vi "Excit_Setup_Wfm.vi"(7 "Excit Number":i32, 8 "error in":errorcluster, 9 "Excit Waveforms File Filter":string, 10 "Excit Waveforms Path":path, 11 "EXCIT Waveforms Inputs":T1={"Excit Form"=enum."Swift", "Amplitude"=100.0, "Start Frequency"=250.0, "End Frequency"=1000.0, "Duration"=800.0, "Sampling Frequency"=5.0, "Swift Factor"=0.5, "Chirp Apodisation"=3.5, "Amplitude 2"=100.0, "Start Frequency 2"=250.0, "End Frequency 2"=350.0} caption="EXCIT Inputs" {"End Frequency 2" min=1.0 max=10000.0; "Start Frequency 2" min=1.0 max=10000.0; "Amplitude 2" min=1.0 max=100.0; "Chirp Apodisation" min=1.0 max=5.0 step=0.1; "Swift Factor" min=0.1 max=3.0 step=0.1; "Sampling Frequency" min=10.0 max=100.0 step=1.0; "Duration" min=1.0 max=1000000.0 step=1.0; "End Frequency" min=1.0 max=10000.0; "Start Frequency" min=1.0 max=10000.0 step=0.1; "Amplitude" min=1.0 max=100.0}) -> (0 "error out":errorcluster caption="sortie d'erreur", 2 "EXCIT Waveforms Inputs":T1={"Excit Form"=enum."Swift", "Amplitude"=100.0, "Start Frequency"=250.0, "End Frequency"=1000.0, "Duration"=800.0, "Sampling Frequency"=5.0, "Swift Factor"=0.5, "Chirp Apodisation"=3.5, "Amplitude 2"=100.0, "Start Frequency 2"=250.0, "End Frequency 2"=350.0} caption="EXCIT Inputs" {"End Frequency 2" min=1.0 max=10000.0; "Start Frequency 2" min=1.0 max=10000.0; "Amplitude 2" min=1.0 max=100.0; "Chirp Apodisation" min=1.0 max=5.0 step=0.1; "Swift Factor" min=0.1 max=3.0 step=0.1; "Sampling Frequency" min=10.0 max=100.0 step=1.0; "Duration" min=1.0 max=1000000.0 step=1.0; "End Frequency" min=1.0 max=10000.0; "Start Frequency" min=1.0 max=10000.0 step=0.1; "Amplitude" min=1.0 max=100.0}, 3 "Waveform Name":string)   [LabVIEW 2017]
doc: "From a start and end value, generates an adiabatic waveform signal of 2000 values (double).\nWrites this waveform into a binary file, in a big-endian format.\nDisplays the written data and the FFT of the signal.\nDefault Path for the generated file is D:\\PIRENEA\\EXCIT_WFMS\n\nAvailable Waveforms : Sinus, Swift, Chirp, Ramp (Up or Down), DoubleRamp (Up-Down or Down-Up)"
uses:
  controls/EXCIT_Waveforms_Inputs.ctl
  <vilib>/Analysis/NI_AALPro.lvlib
panel:
  out "Waveform Name":string
  in  "OK":bool
  out "Excitation FFT":cluster{dbl[], "Power Spectrum (V^2 rms)":dbl[]}(graph)
  out "Excitation Signal":T2(graph)
  out "FIFO used":i32
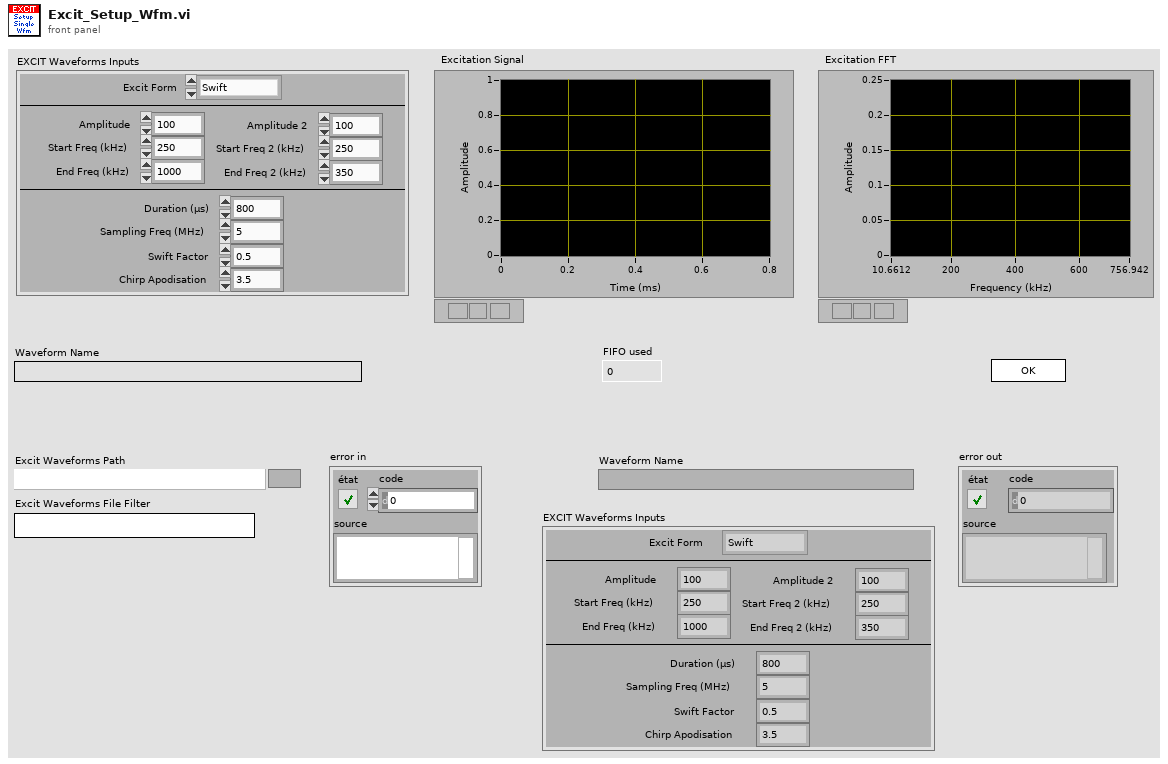
[diagram p1: front panel]
types:
  T1 = typedef "EXCIT_Waveforms_Inputs.ctl" = cluster{"Excit Form":enum16{"Sinus", "Chirp", "Swift", "TwoSwift", "Ramp"}, "Amplitude":dbl, "Start Frequency":dbl, "End Frequency":dbl, "Duration":dbl, "Sampling Frequency":dbl, "Swift Factor":dbl, "Chirp Apodisation":dbl, "Amplitude 2":dbl, "Start Frequency 2":dbl, "End Frequency 2":dbl}
  T2 = cluster{"X Time":dbl[], "Signal Excitation":dbl[]}
  T3 = enum16{"open", "replace", "create", "open or create", "replace or create", "replace or create with confirmation"}
  T4 = enum16{"big-endian, network order", "native, host order", "little-endian"}
  T5 = enum16{"Sinus", "Chirp", "Swift", "TwoSwift", "Ramp"}
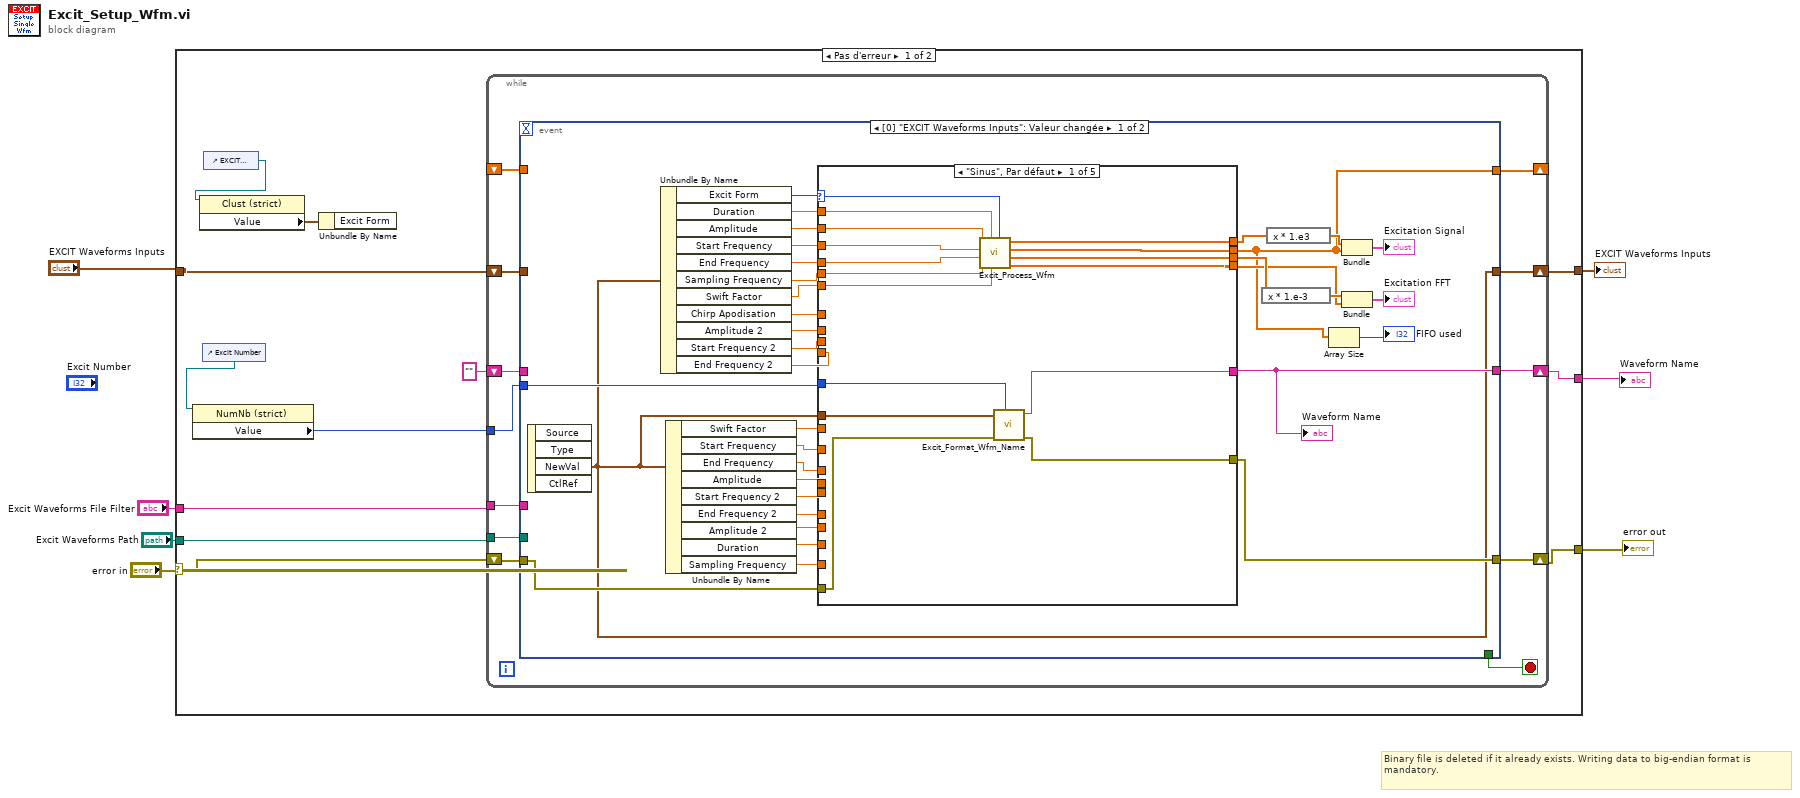
[diagram p0: block diagram]
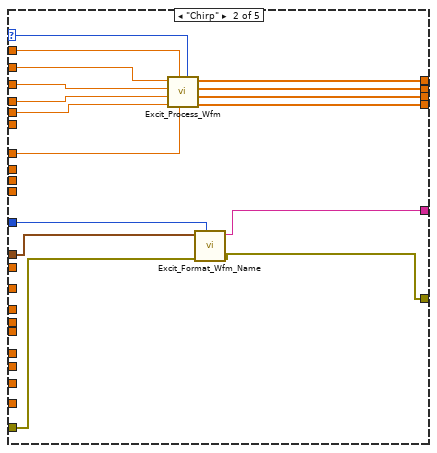
[diagram p2: hidden frame]
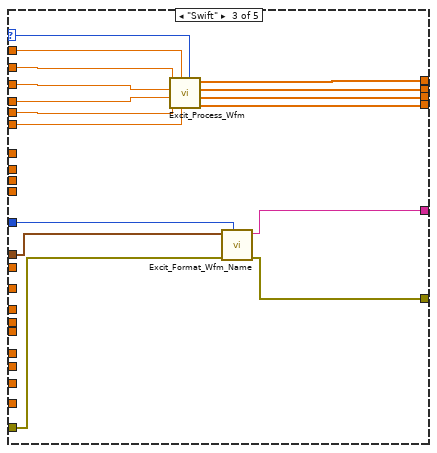
[diagram p3: hidden frame]
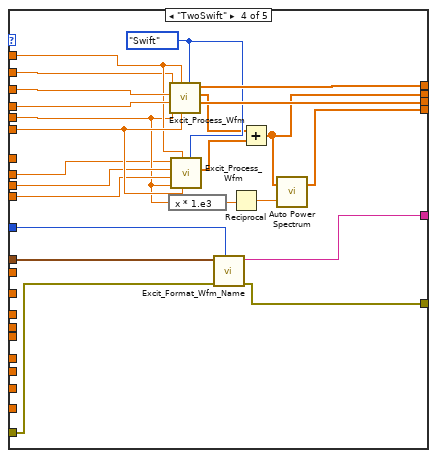
[diagram p4: hidden frame]
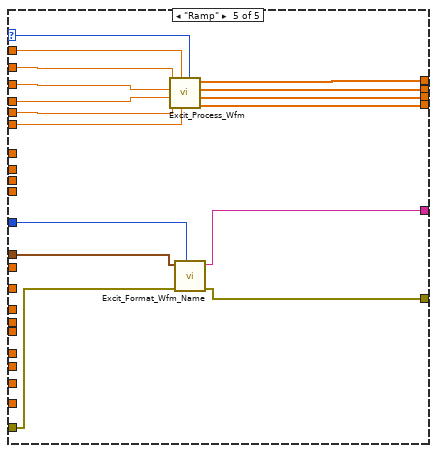
[diagram p5: hidden frame]
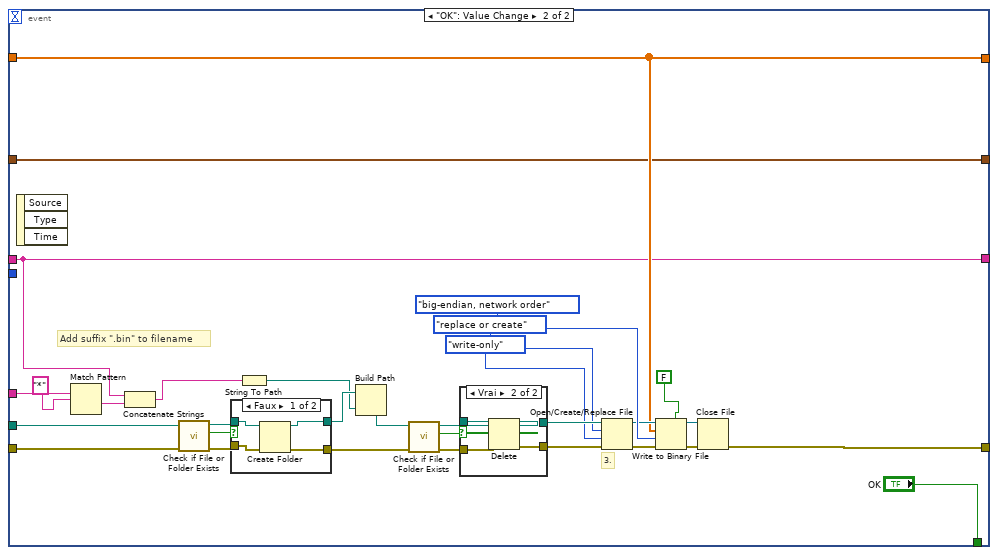
[diagram p6: hidden frame]
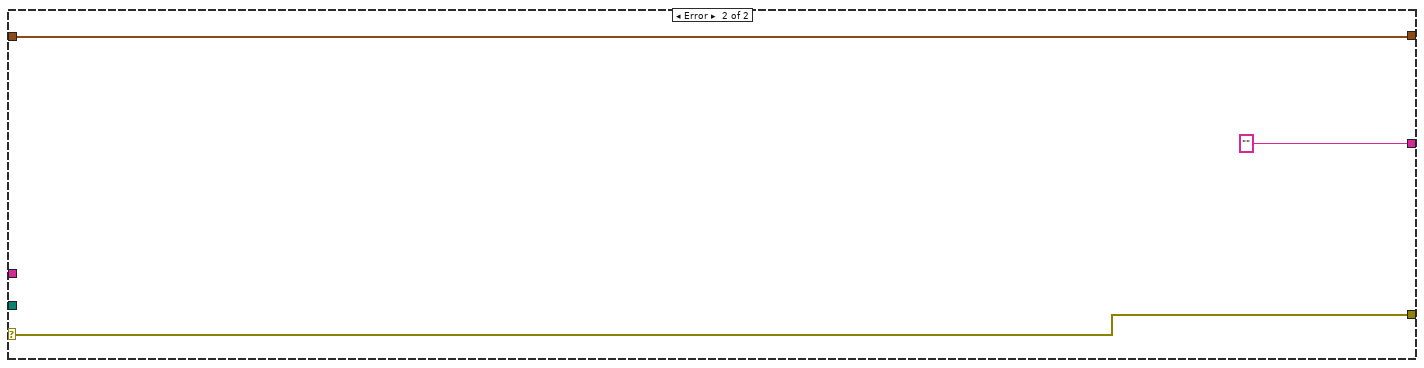
[diagram p9: hidden frame]
diagram:
  # "Binary file is deleted if it already exists. Writing data to big-endian format is mandatory."
  n1 = case shown="Pas d'erreur" "error in" {
    selector: "error in" -> [w10 w198]
    tunnel: [w19 w198] -> w7
    tunnel: "Excit Waveforms Path" -> [w18 _]
    tunnel: [w17 ""] -> w4
    tunnel: "Excit Waveforms File Filter" -> [w16 _]
    tunnel: "EXCIT Waveforms Inputs" -> [w14 w197]
    tunnel: [w13 w197] -> w1
    frame No Error {
      n2 = control-ref of="Excit Number"() -> (w12:refnum<vi>)
      n3 = property class="NumNb (strict)"(reference=w12) -> ("Value"=w11:i32)  [unwired: 1 in, 2 out]
      n4 = control-ref of="EXCIT Waveforms Inputs"() -> (w9:refnum<vi>)
      n5 = property class="Clust (strict)"(reference=w9) -> ("Value"=w8:T1)  [unwired: 1 in, 2 out]
      n6 = Unbundle By Name(w8) -> ()  [unwired: 1 out]
      n7 = while {
        tunnel: w18 -> [w25]
        shift-right: [w24] -> w19
        shift-left: w10 -> [w31]
        shift-right: [w29] -> _
        shift-left: _ -> [w27]
        shift-right: [w28] -> w17
        shift-left: "" -> [w26]
        tunnel: w16 -> [w23]
        shift-right: [w21] -> w13
        shift-left: w14 -> [w22]
        tunnel: w11 -> [w20]
        stop <- w30 stop-if-true
        n8 = event shown="[0] \"EXCIT Waveforms Inputs\": Valeur changée" {
          selector: _ -> [_ _]
          dyn-events: _ -> [_ _]
          timeout: _ -> [_ _]
          tunnel: [w36 w160] -> w24
          tunnel: w31 -> [w38 w162]
          tunnel: [_ "OK"] -> w30
          tunnel: [w37 w159] -> w29
          tunnel: [w35 w155] -> w28
          tunnel: w27 -> [_ w159]
          tunnel: w26 -> [_ w155]
          tunnel: w25 -> [_ w161]
          tunnel: w23 -> [_ w158]
          tunnel: w22 -> [_ w153]
          tunnel: [w32 w153] -> w21
          tunnel: w20 -> [w34 _]
          event Value Change {
            n9 = event-data() -> ("NewVal"=w32:T1)  [unwired: 1 in, 3 out]
            n10 = Unbundle By Name(w32) -> ("Excit Form"=w62:T5, "Duration"=w61:dbl, "Amplitude"=w60:dbl, "Start Frequency"=w59:dbl, "End Frequency"=w58:dbl, "Sampling Frequency"=w57:dbl, "Swift Factor"=w56:dbl, "Chirp Apodisation"=w55:dbl, "Amplitude 2"=w49:dbl, "Start Frequency 2"=w48:dbl, "End Frequency 2"=w47:dbl)
            n11 = Unbundle By Name(w32) -> ("Swift Factor"=w33:dbl, "Start Frequency"=w46:dbl, "End Frequency"=w45:dbl, "Amplitude"=w44:dbl, "Start Frequency 2"=w39:dbl, "End Frequency 2"=w43:dbl, "Amplitude 2"=w42:dbl, "Duration"=w41:dbl, "Sampling Frequency"=w40:dbl)
            n12 = case shown="\"Sinus\", Par défaut" w62 {
              selector: w62 -> [w80 w97 w107 _ w142]
              tunnel: w55 -> [_ w91 _ _ _]
              tunnel: w61 -> [w81 w96 w108 w122 w147]
              tunnel: w60 -> [w79 w95 w109 w120 w148]
              tunnel: w59 -> [w78 w94 w110 w126 w149]
              tunnel: w58 -> [w77 w93 w111 w125 w150]
              tunnel: w57 -> [w76 w92 w112 w121 w151]
              tunnel: w56 -> [w75 _ w113 w133 w152]
              tunnel: [w74 w90 w106 w136 w146] -> w54
              tunnel: [w73 w89 w105 w129 w145] -> w37
              tunnel: [w72 w88 w104 w135 w144] -> w52
              tunnel: [w71 w87 w103 w127 w143] -> w51
              tunnel: w49 -> [_ _ _ w119 _]
              tunnel: w48 -> [_ _ _ w124 _]
              tunnel: w47 -> [_ _ _ w123 _]
              tunnel: [w67 w82 w99 w114 w139] -> w36
              tunnel: [w66 w83 w98 w115 w137] -> w35
              tunnel: w46 -> [_ _ _ _ _]
              tunnel: w45 -> [_ _ _ _ _]
              tunnel: w44 -> [_ _ _ _ _]
              tunnel: w43 -> [_ _ _ _ _]
              tunnel: w42 -> [_ _ _ _ _]
              tunnel: w41 -> [_ _ _ _ _]
              tunnel: w40 -> [_ _ _ _ _]
              tunnel: w39 -> [_ _ _ _ _]
              tunnel: w38 -> [w68 w84 w100 w116 w140]
              tunnel: w34 -> [w70 w86 w102 w118 w138]
              tunnel: w33 -> [_ _ _ _ _]
              tunnel: w32 -> [w69 w85 w101 w117 w141]
              frame "Sinus", Default {
                n13 = call "Excit_Process_Wfm.vi"("Excit Form"=w80, "Factor"=w75, "Duration (µs)"=w81, "Sampling Frequency (MHz)"=w76, "End Frequency (kHz)"=w77, "Start Frequency (kHz)"=w78, "Amplitude (%)"=w79) -> ("FFT Excitation"=w71:dbl[], "X Freq"=w72:dbl[], "Signal Excitation"=w73:dbl[], "X Time"=w74:dbl[])
                n14 = call "Excit_Format_Wfm_Name.vi"("Excit Number"=w70, "error in"=w68, "EXCIT Waveforms Inputs"=w69) -> ("error out"=w67:errorcluster, "Waveform Name"=w66:string)  [unwired: 7 in]
              }
              frame "Chirp" {
                n15 = call "Excit_Process_Wfm.vi"("Excit Form"=w97, "Factor"=w91, "Duration (µs)"=w96, "Sampling Frequency (MHz)"=w92, "End Frequency (kHz)"=w93, "Start Frequency (kHz)"=w94, "Amplitude (%)"=w95) -> ("FFT Excitation"=w87:dbl[], "X Freq"=w88:dbl[], "Signal Excitation"=w89:dbl[], "X Time"=w90:dbl[])
                n16 = call "Excit_Format_Wfm_Name.vi"("Excit Number"=w86, "error in"=w84, "EXCIT Waveforms Inputs"=w85) -> ("error out"=w82:errorcluster, "Waveform Name"=w83:string)  [unwired: 7 in]
              }
              frame "Swift" {
                n17 = call "Excit_Process_Wfm.vi"("Excit Form"=w107, "Factor"=w113, "Duration (µs)"=w108, "Sampling Frequency (MHz)"=w112, "End Frequency (kHz)"=w111, "Start Frequency (kHz)"=w110, "Amplitude (%)"=w109) -> ("FFT Excitation"=w103:dbl[], "X Freq"=w104:dbl[], "Signal Excitation"=w105:dbl[], "X Time"=w106:dbl[])
                n18 = call "Excit_Format_Wfm_Name.vi"("Excit Number"=w102, "error in"=w100, "EXCIT Waveforms Inputs"=w101) -> ("error out"=w99:errorcluster, "Waveform Name"=w98:string)  [unwired: 7 in]
              }
              frame "TwoSwift" {
                w134 = T5."Swift" ("Excit Form")
                n19 = expression code="x * 1.e3"(w121) -> (w130:dbl)
                n20 = call "Excit_Process_Wfm.vi"("Excit Form"=w134, "Factor"=w133, "Duration (µs)"=w122, "Sampling Frequency (MHz)"=w121, "End Frequency (kHz)"=w125, "Start Frequency (kHz)"=w126, "Amplitude (%)"=w120) -> ("X Freq"=w135:dbl[], "Signal Excitation"=w132:dbl[], "X Time"=w136:dbl[])  [unwired: 1 out]
                n21 = call "Excit_Process_Wfm.vi"("Excit Form"=w134, "Factor"=w133, "Duration (µs)"=w122, "Sampling Frequency (MHz)"=w121, "End Frequency (kHz)"=w123, "Start Frequency (kHz)"=w124, "Amplitude (%)"=w119) -> ("Signal Excitation"=w131:dbl[])  [unwired: 3 out]
                n22 = call "Excit_Format_Wfm_Name.vi"("Excit Number"=w118, "error in"=w116, "EXCIT Waveforms Inputs"=w117) -> ("error out"=w114:errorcluster, "Waveform Name"=w115:string)  [unwired: 7 in]
                n23 = Reciprocal(x=w130) -> (1/x=w128:dbl)
                n24 = Add(x=w132, y=w131) -> (x+y=w129:dbl[])
                n25 = call <vilib>:"Auto Power Spectrum.vi"("dt"=w128, "Signal (V)"=w129) -> ("Power Spectrum (V^2 rms)"=w127:dbl[])  [unwired: 1 out]
              }
              frame "Ramp" {
                n26 = call "Excit_Process_Wfm.vi"("Excit Form"=w142, "Factor"=w152, "Duration (µs)"=w147, "Sampling Frequency (MHz)"=w151, "End Frequency (kHz)"=w150, "Start Frequency (kHz)"=w149, "Amplitude (%)"=w148) -> ("FFT Excitation"=w143:dbl[], "X Freq"=w144:dbl[], "Signal Excitation"=w145:dbl[], "X Time"=w146:dbl[])
                n27 = call "Excit_Format_Wfm_Name.vi"("Excit Number"=w138, "error in"=w140, "EXCIT Waveforms Inputs"=w141) -> ("error out"=w139:errorcluster, "Waveform Name"=w137:string)  [unwired: 7 in]
              }
            }
            "Waveform Name" <- w35
            n28 = expression code="x * 1.e-3"(w52) -> (w63:dbl[])
            n29 = expression code="x * 1.e3"(w54) -> (w64:dbl[])
            n30 = Array Size(array=w37) -> (size(s)=→"FIFO used":i32)
            n31 = Bundle("X Time"=w64, "Signal Excitation"=w37) -> (→"Excitation Signal":T2)  [unwired: 1 in]
            n32 = Bundle("X Freq"=w63, "FFT Excitation"=w51) -> (→"Excitation FFT":cluster{"X Freq":dbl[], "FFT Excitation":dbl[]})  [unwired: 1 in]
          }
          event "OK": Value Change {
            # "Add suffix \".bin\" to filename"
            # "3."
            n33 = event-data() -> ()  [unwired: 1 in, 3 out]
            n34 = Match Pattern(string=w158, regular expression="*" ("expression régulière")) -> (after substring=w156:string)  [unwired: 1 in, 3 out]
            n35 = Concatenate Strings(w155, w156) -> (w154:string)
            n36 = call <vilib>:"Check if File or Folder Exists.vi"("error in (no error)"=w162, "path"=w161) -> ("error out"=w180:errorcluster, "file or folder exists?"=w178:bool, "dup path"=w179:path)  [unwired: 7 in]
            n37 = case shown="Faux" w178 {
              tunnel: w179 -> [w193 w195]
              tunnel: [w192 w195] -> w181
              tunnel: w180 -> [w191 w194]
              tunnel: [w190 w194] -> w182
              frame False {
                n38 = Create Folder(path (use dialog)=w193, error in=w191) -> (created path=w192:path, error out=w190:errorcluster)  [unwired: 1 in, 1 out]
              }
              frame True {
              }
            }
            n39 = String To Path(string=w154) -> (path=w171:path)
            n40 = Build Path(base path=w181, name or relative path=w171) -> (appended path=w175:path)
            n41 = call <vilib>:"Check if File or Folder Exists.vi"("error in (no error)"=w182, "path"=w175) -> ("error out"=w174:errorcluster, "file or folder exists?"=w173:bool, "dup path"=w172:path)  [unwired: 7 in]
            n42 = case shown="Vrai" w173 {
              tunnel: w172 -> [w185 w189]
              tunnel: w174 -> [w184 w188]
              tunnel: [w185 w187] -> w176
              tunnel: [w184 w186] -> w177
              frame False {
              }
              frame True {
                n43 = Delete(path (use dialog)=w189, error in=w188) -> (deleted path=w187:path, error out=w186:errorcluster)  [unwired: 3 in, 1 out]
              }
            }
            n44 = Open/Create/Replace File(file path (use dialog)=w176, error in=w177, operation (0:open)=T3."replace or create", access (0:read/write)=enum16{"read/write", "read-only", "write-only"}."write-only") -> (refnum out=w166:refnum<file>, error out=w165:errorcluster)  [unwired: 2 in, 1 out]
            n45 = Write to Binary File(file (use dialog)=w166, data=w159, error in=w165, 5:FALSE ("prepend array or string size? (T)"), 9:T4."big-endian, network order" ("byte order")) -> (refnum out=w163:refnum<file>, error out=w164:errorcluster)  [unwired: 1 in, 1 out]
            n46 = Close File(refnum=w163, error in=w164) -> (error out=w160:errorcluster)  [unwired: 1 out]
          }
        }
      }
    }
    frame Error {
    }
  }
  "error out" <- w7
  "Waveform Name" <- w4
  "EXCIT Waveforms Inputs" <- w1
